vi "测验程序1.vi"() -> ()   [LabVIEW 2017]
uses:
  <vilib>/Platform/TimedLoop/XDataNode/timing_clust.ctl
  <vilib>/Platform/TimedLoop/XDataNode/nitl_modes.ctl
  <vilib>/Platform/TimedLoop/XDataNode/wakeup.ctl
  <vilib>/myRIO/Common/Instrument Driver Framework/myRIO v1.0/UART/vis/myRIO v1.0 Close UART.vi
  <vilib>/FPGAPlugInAG/myRIO-1900/niLvFpga_Open_myRIO-1900.vi
  <vilib>/rvi/interface/common/dynamic/niFpgaDynamicAddResources.vi
  <vilib>/myRIO/Common/Instrument Driver Framework/Utilities/vis/FPGA Ref Manager.vi
  <vilib>/Utility/error.llb/Error Cluster From Error Code.vi
  <vilib>/myRIO/Common/Instrument Driver Framework/Utilities/vis/Ref Counter.vi
  <vilib>/FPGAPlugInAG/Dynamic/niLvFpga_Close_Dynamic.vi
  <vilib>/myRIO/Common/Instrument Driver Framework/myRIO v1.0/myRIO v1.0 Reset FPGA.vi
  <vilib>/myRIO/Common/Instrument Driver Framework/myRIO v1.0/IRQ/vis/myRIO v1.0 IRQ Info FGV.vi
  <vilib>/myRIO/Common/Instrument Driver Framework/myRIO v1.0/IRQ/vis/myRIO v1.0 Timer IRQ Info FGV.vi
  <vilib>/myRIO/Common/Instrument Driver Framework/myRIO v1.0/IRQ/vis/myRIO v1.0 ISR Agent.vi
  <vilib>/Platform/TimedLoop/XDataNode/XDataNode.xnode
  <vilib>/rvi/interface/nirviOpenFPGA/nirviOpenFPGA.xnode
  <vilib>/rvi/interface/nirviCloseFPGA/nirviCloseFPGA.xnode
  <vilib>/Platform/TimedLoop/XDataNode/XDNodeRunTimeDep.lvlib
  <vilib>/myRIO/Instrument Drivers/Utilities/Utilities.lvlib
panel:
  out "当前步态":u16
  out "超声波":u32[](array[numeric])
  in  "平移距离":i32
  in  "停止":bool
  in  "90":i32
  in  "360":i32
  in  "开始":bool
  in  "初始步态":u16(ring) items=["等待", "90", "暂停1s", "360", "短暂停", "前", "短暂停", "后", "短暂停", "左", "短暂停", "右", "短暂停"]
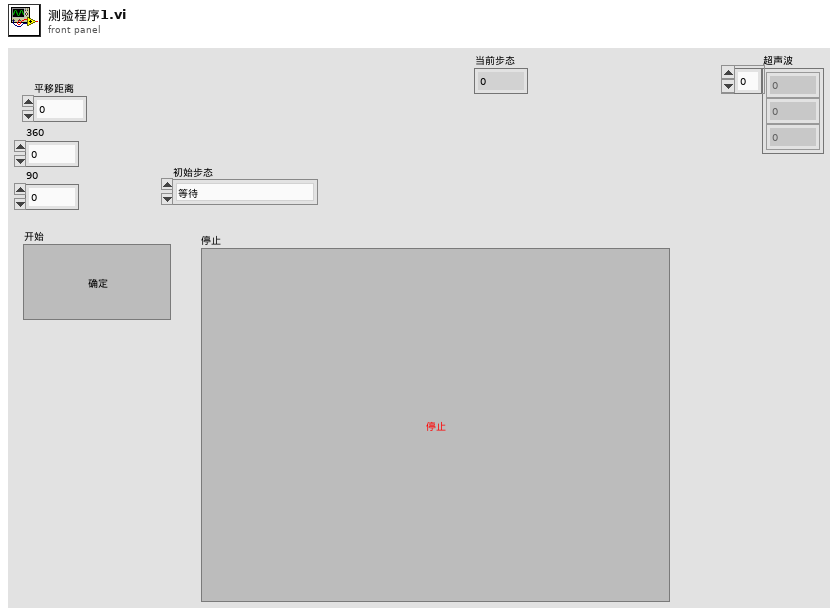
[diagram p1: front panel]
types:
  T1 = typedef "XDNodeRunTimeDep.lvlib/timing_clust.ctl" = cluster{"Expected End [f-1]":u64, "Actual End [f-1]":u64, "Finished Late? [f-1]":bool, "Expected End [i-1]":u64, "Actual End [i-1]":u64, "Finished Late? [i-1]":bool, "Expected Start [i]":u64, "Actual Start [i]":u64, "Expected Start [f]":u64, "Actual Start [f]":u64, "Source Name":string, "Structure Name":string, "Period":i64, "Deadline":i64, "Offset":i64, "Start":i64, "Priority":i32, "Timeout":i32, "Mode":T2, "Wakeup Reason":T3, "Error":errorcluster, "Source Type":string, "Secondary Source Type":string, "Global End Time":u64, "Global Start Time":u64, "Frame Duration":u64, "Iteration Duration":u64, "Assigned CPU":i32, "I/O Scan Engine Mode":u32}
  T2 = typedef "XDNodeRunTimeDep.lvlib/nitl_modes.ctl" = enum32{"No Change", "Process missed periods, maintain original phase", "Discard missed periods, maintain original phase", "Process missed periods, ignore original phase", "Discard missed periods, ignore original phase"}
  T3 = typedef "XDNodeRunTimeDep.lvlib/wakeup.ctl" = enum32{"Normal", "Aborted", "Asynchronous wakeup", "Timing source error", "Timed loop error", "Timeout"}
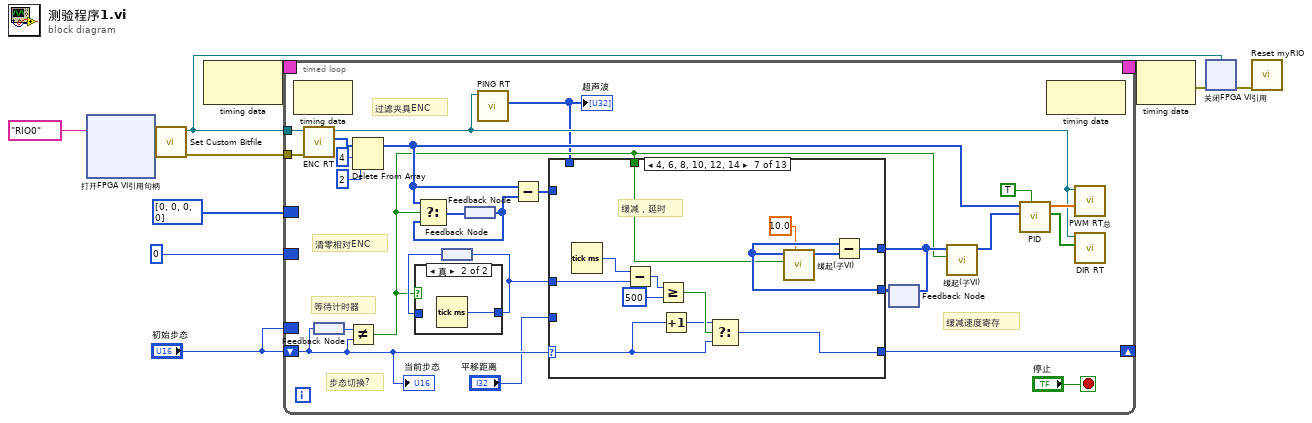
[diagram p0: block diagram]
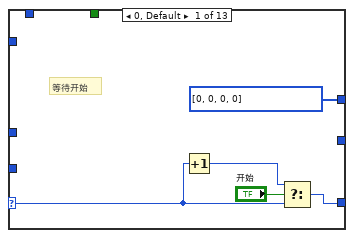
[diagram p3: hidden frame]
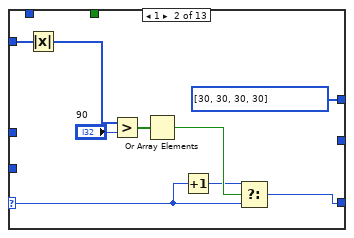
[diagram p4: hidden frame]
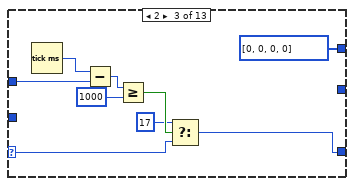
[diagram p5: hidden frame]
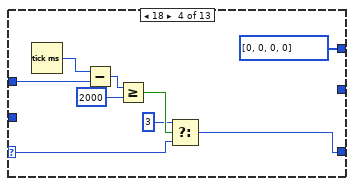
[diagram p6: hidden frame]
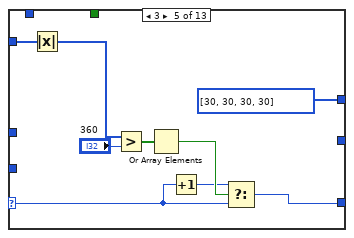
[diagram p7: hidden frame]
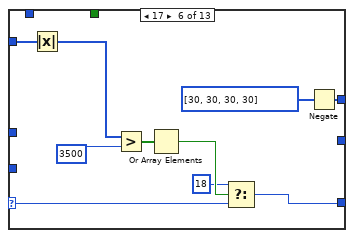
[diagram p8: hidden frame]
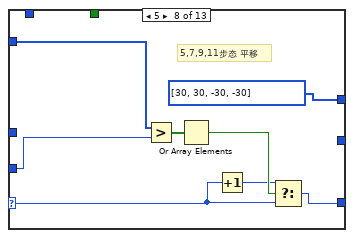
[diagram p9: hidden frame]
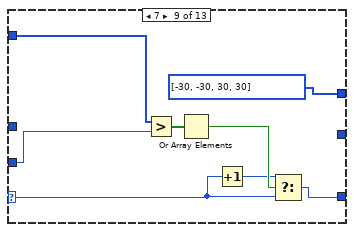
[diagram p10: hidden frame]
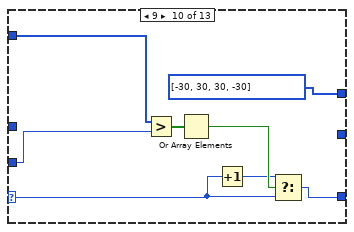
[diagram p11: hidden frame]
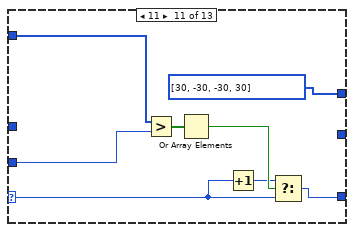
[diagram p12: hidden frame]
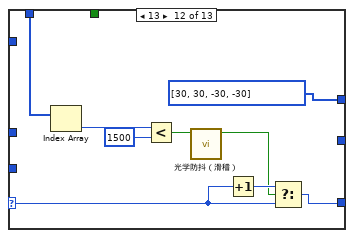
[diagram p13: hidden frame]
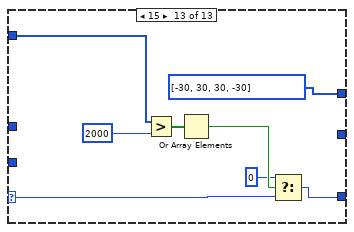
[diagram p14: hidden frame]
diagram:
  n1 = xnode "打开FPGA VI引用句柄"("资源名称"=tag "RIO0") -> ("FPGA VI引用输出"=w6:refnum<k20>, "错误输出"=w5:errorcluster)  [unwired: 1 in]
  n2 = call <vilib>:"Set Custom Bitfile.vi"("error in (no error)"=w5, "Custom FPGA Reference In"=w6) -> ("error out"=w4:errorcluster, "Custom FPGA Reference Out"=w1:refnum<k20>)  [unwired: 8 in]
  n3 = node-c288() -> (w12:T1)  [unwired: 1 in]
  n4 = timed-loop {
    timing: w12 -> [_]
    timing-out: [_] -> w11
    shift-right: [w35] -> _
    shift-left: "初始步态" -> [w33]
    border: "初始步态" -> [_]
    border: i32[] [0, 0, 0, 0] ("ENC") -> [_]
    tunnel: w4 -> [w30]
    tunnel: w1 -> [w15]
    border: u32 0 ("millisecond timer value") -> [_]
    stop <- "停止" stop-if-true
    # "缓减速度寄存"
    # "步态切换?"
    # "等待计时器"
    # "清零相对ENC"
    # "过滤夹具ENC"
    n5 = node-c288() -> ()  [unwired: 1 in, 1 out]
    n6 = call "ENC RT.vi"("错误输入（无错误）"=w30, "Custom FPGA Reference Out"=w15) -> ("ENC"=w28:i32[], "FPGA VI引用输出"=w14:refnum<k20>)  [unwired: 7 in, 1 out]
    n7 = feedback-in #1(w33) -> ()
    n8 = feedback #1() -> (w34:u16)
    n9 = Not Equal?(x=w34, y=w33) -> (x != y?=w16:bool)
    n10 = Delete From Array(array=w28, length=2 ("长度"), index=4 ("索引")) -> (array with subset deleted=w23:i32[])  [unwired: 1 out]
    n11 = feedback #2() -> (w22:u32)
    n12 = case shown="真" w16 {
      tunnel: [w38 w39] -> w21
      tunnel: w22 -> [w38 _]
      frame False {
      }
      frame True {
        n13 = Tick Count (ms)() -> (millisecond timer value=w39:u32)
      }
    }
    n14 = feedback-in #2(w21) -> ()
    n15 = feedback #3() -> (w24:i32[])
    n16 = Select(t=w23, s=w16, f=w24) -> (s? t:f=w32:i32[])
    n17 = feedback-in #3(w32) -> ()
    n18 = call "PING RT.vi"("引用句柄输入"=w14) -> ("PING"=w13:u32[])  [unwired: 8 in, 2 out]
    "超声波" <- w13
    n19 = Subtract(x=w23, y=w24) -> (x-y=w25:i32[])
    n20 = feedback #4() -> (w17:i32[])  [unwired: 1 in]
    n21 = case shown="4, 6, 8, 10, 12, 14" w33 {
      selector: w33 -> [w41 w46 w56 w65 w73 w84 w97 w106 w114 w122 w128 w141 w148]
      tunnel: [w43 w47 w55 w64 w74 w85 w96 w105 w113 w121 w131 w143 w147] -> w35
      tunnel: [i32[] [0, 0, 0, 0] ("SET") i32[] [30, 30, 30, 30] ("SET") i32[] [0, 0, 0, 0] ("SET") i32[] [0, 0, 0, 0] ("SET") i32[] [30, 30, 30, 30] ("SET") w83 w92 i32[] [30, 30, -30, -30] ("SET") i32[] [-30, -30, 30, 30] ("SET") i32[] [-30, 30, 30, -30] ("SET") i32[] [30, -30, -30, 30] ("SET") i32[] [30, 30, -30, -30] ("SET") i32[] [-30, 30, 30, -30] ("SET")] -> w18
      tunnel: w25 -> [_ w52 _ _ w76 w87 _ w107 w115 w123 w132 _ w149]
      tunnel: w21 -> [_ _ w60 w69 _ _ w102 _ _ _ _ _ _]
      tunnel: "平移距离" -> [_ _ _ _ _ _ _ w104 w112 w120 w130 _ _]
      tunnel: w17 -> [_ _ _ _ _ _ w94 _ _ _ _ _ _]
      tunnel: w16 -> [_ _ _ _ _ _ w93 _ _ _ _ _ _]
      tunnel: w13 -> [_ _ _ _ _ _ _ _ _ _ _ w139 _]
      frame 0, Default {
        # "等待开始"
        n22 = Increment(x=w41) -> (x+1=w40:u16)
        n23 = Select(t=w40, s="开始", f=w41) -> (s? t:f=w43:u16)
      }
      frame 1 {
        n24 = Absolute Value(x=w52) -> (abs(x)=w51:i32[])
        n25 = Greater?(x=w51, y="90") -> (0:w49:bool[])
        n26 = Or Array Elements(Boolean array=w49) -> (logical OR=w48:bool)
        n27 = Increment(x=w46) -> (x+1=w45:u16)
        n28 = Select(t=w45, s=w48, f=w46) -> (s? t:f=w47:u16)
      }
      frame 2 {
        n29 = Tick Count (ms)() -> (millisecond timer value=w61:u32)
        n30 = Subtract(x=w61, y=w60) -> (x-y=w59:u32)
        n31 = Greater Or Equal?(x=w59, y=u32 1000) -> (x >= y?=w57:bool)
        n32 = Select(t=u16 17, s=w57, f=w56) -> (s? t:f=w55:u16)
      }
      frame 18 {
        n33 = Tick Count (ms)() -> (millisecond timer value=w70:u32)
        n34 = Subtract(x=w70, y=w69) -> (x-y=w68:u32)
        n35 = Greater Or Equal?(x=w68, y=u32 2000) -> (x >= y?=w66:bool)
        n36 = Select(t=u16 3, s=w66, f=w65) -> (s? t:f=w64:u16)
      }
      frame 3 {
        n37 = Absolute Value(x=w76) -> (abs(x)=w79:i32[])
        n38 = Greater?(x=w79, y="360") -> (0:w77:bool[])
        n39 = Or Array Elements(Boolean array=w77) -> (logical OR=w75:bool)
        n40 = Increment(x=w73) -> (x+1=w72:u16)
        n41 = Select(t=w72, s=w75, f=w73) -> (s? t:f=w74:u16)
      }
      frame 17 {
        n42 = Absolute Value(x=w87) -> (abs(x)=w89:i32[])
        n43 = Greater?(x=w89, y=3500) -> (0:w88:bool[])
        n44 = Or Array Elements(Boolean array=w88) -> (logical OR=w86:bool)
        n45 = Select(t=u16 18, s=w86, f=w84) -> (s? t:f=w85:u16)
        n46 = Negate(x=i32[] [30, 30, 30, 30] ("SET")) -> (-x=w83:i32[])
      }
      frame 4, 6, 8, 10, 12, 14 {
        # "缓减，延时"
        n47 = Tick Count (ms)() -> (millisecond timer value=w103:u32)
        n48 = Subtract(x=w103, y=w102) -> (x-y=w101:u32)
        n49 = Greater Or Equal?(x=w101, y=u32 500) -> (x >= y?=w99:bool)
        n50 = Increment(x=w97) -> (x+1=w98:u16)
        n51 = Select(t=w98, s=w99, f=w97) -> (s? t:f=w96:u16)
        n52 = call "缓起(子VI).vi"("循环数(100)"=10.0, "缓起清零"=w93, "输入"=w94) -> ("输出"=w95:i32[])  [unwired: 8 in]
        n53 = Subtract ("减")(x=w94, y=w95) -> (x-y=w92:i32[])
      }
      frame 5 {
        # "5,7,9,11步态 平移"
        n54 = Greater?(x=w107, y=w104) -> (0:w110:bool[])
        n55 = Or Array Elements(Boolean array=w110) -> (logical OR=w109:bool)
        n56 = Increment(x=w106) -> (x+1=w108:u16)
        n57 = Select(t=w108, s=w109, f=w106) -> (s? t:f=w105:u16)
      }
      frame 7 {
        n58 = Greater?(x=w115, y=w112) -> (0:w118:bool[])
        n59 = Or Array Elements(Boolean array=w118) -> (logical OR=w117:bool)
        n60 = Increment(x=w114) -> (x+1=w116:u16)
        n61 = Select(t=w116, s=w117, f=w114) -> (s? t:f=w113:u16)
      }
      frame 9 {
        n62 = Greater?(x=w123, y=w120) -> (0:w126:bool[])
        n63 = Or Array Elements(Boolean array=w126) -> (logical OR=w125:bool)
        n64 = Increment(x=w122) -> (x+1=w124:u16)
        n65 = Select(t=w124, s=w125, f=w122) -> (s? t:f=w121:u16)
      }
      frame 11 {
        n66 = Greater?(x=w132, y=w130) -> (0:w134:bool[])
        n67 = Or Array Elements(Boolean array=w134) -> (logical OR=w133:bool)
        n68 = Increment(x=w128) -> (x+1=w129:u16)
        n69 = Select(t=w129, s=w133, f=w128) -> (s? t:f=w131:u16)
      }
      frame 13 {
        n70 = Index Array(array=w139) -> (element=w138:u32)  [unwired: 1 in]
        n71 = Less?(x=w138, y=u32 1500) -> (x < y?=w137:bool)
        n72 = call "光学防抖（滑稽）.vi"("布尔输入"=w137) -> ("布尔输出"=w136:bool)  [unwired: 10 in]
        n73 = Increment(x=w141) -> (x+1=w142:u16)
        n74 = Select(t=w142, s=w136, f=w141) -> (s? t:f=w143:u16)
      }
      frame 15 {
        n75 = Greater?(x=w149, y=2000 ("长度")) -> (0:w151:bool[])
        n76 = Or Array Elements(Boolean array=w151) -> (logical OR=w150:bool)
        n77 = Select(t=u16 0, s=w150, f=w148) -> (s? t:f=w147:u16)
      }
    }
    n78 = feedback-in #4(w18) -> ()
    n79 = call "缓起(子VI).vi"("缓起清零"=w16, "输入"=w18) -> ("输出"=w19:i32[])  [unwired: 9 in]
    n80 = call "PID.vi"("继电器"=TRUE, "SET"=w19, "ENC"=w23) -> ("DIR"=w36:bool[], "PWM"=w37:dbl[])  [unwired: 7 in]
    n81 = node-c288() -> ()  [unwired: 1 in, 1 out]
    n82 = call "PWM RT总.vi"("PWM"=w37, "Custom FPGA Reference Out"=w14) -> ()  [unwired: 8 in, 2 out]
    n83 = call "DIR RT.vi"("DIR"=w36, "Custom FPGA Reference Out"=w14) -> ()  [unwired: 8 in, 2 out]
    "当前步态" <- w33
  }
  n84 = node-c288(w11) -> (w8:errorcluster)
  n85 = xnode "关闭FPGA VI引用"("FPGA VI引用输入"=w1, "错误输入"=w8) -> ("错误输出"=w7:errorcluster)
  n86 = call <vilib>:"Reset myRIO.vi"("error in (no error)"=w7) -> ()  [unwired: 10 in, 1 out]
